vi "Get Vim-formation.vi"(8 "error in (no error)":errorcluster, 9 "ProjectItem Refnum":refnum<vi>, 10 "Path":path, 11 "Map in":map{path, T1}(c390)) -> (0 "error out":errorcluster, 3 "Map out":map{path, T1}(c390))   [LabVIEW 2020, in "vim-liner.lvlib"]
uses:
  vim-liner.lvlib
  vim-formation.ctl
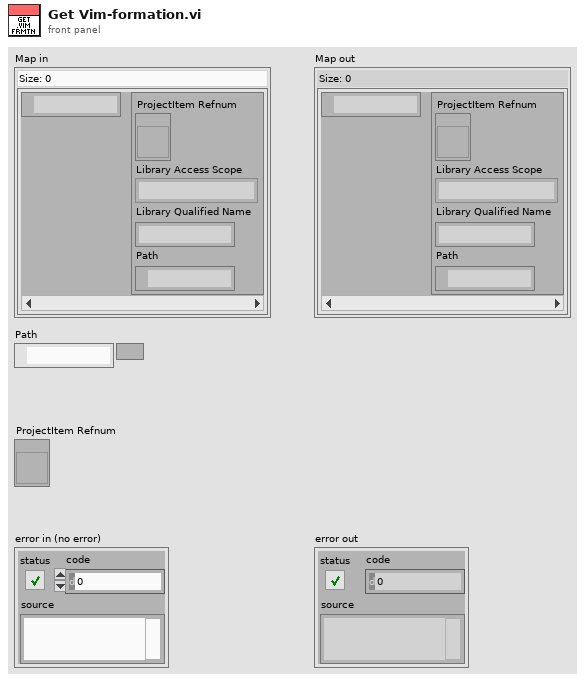
[diagram p1: front panel]
types:
  T1 = typedef "vim-liner.lvlib/vim-formation.ctl" = cluster{"ProjectItem Refnum":refnum<vi>, "Library Access Scope":enum32{"invalid scope", "public", "private", "protected", "community"}, "Library Qualified Name":string, "Path":path}
  T2 = enum32{"invalid scope", "public", "private", "protected", "community"}
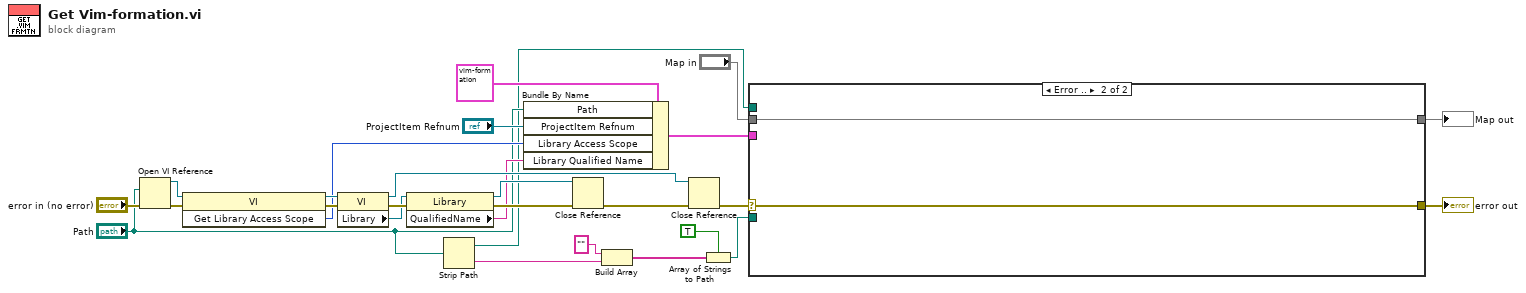
[diagram p0: block diagram]
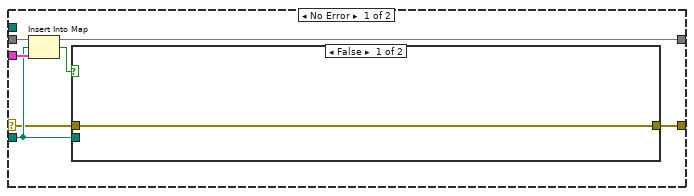
[diagram p2: hidden frame]
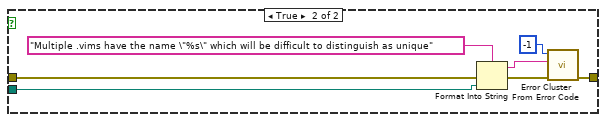
[diagram p3: hidden frame]
diagram:
  n1 = Open VI Reference(vi path="Path", error in (no error)="error in (no error)") -> (vi reference=w18:refnum<vi>, error out=w17:errorcluster)  [unwired: 4 in]
  n2 = invoke class="VI" method="Get Library Access Scope"(reference=w18, error in=w17) -> (reference out=w19:refnum<vi>, error out=w20:errorcluster, "Get Library Access Scope"=w10:T2)  [unwired: 1 in]
  n3 = property class="VI"(reference=w19, error in=w20) -> (reference out=w26:refnum<vi>, error out=w22:errorcluster, "Library"=w21:refnum<vi>)
  n4 = property class="Library"(reference=w21, error in=w22) -> (reference out=w24:refnum<vi>, error out=w23:errorcluster, "QualifiedName"=w9:string)
  n5 = Strip Path(path="Path") -> (stripped path=w7:path, name=w6:string)
  n6 = Bundle By Name(cluster=T1 {"ProjectItem Refnum"=refnum, "Library Access Scope"=enum."invalid scope", "Library Qualified Name"="", "Path"=path ""} (".vim"), "Path"="Path", "ProjectItem Refnum"="ProjectItem Refnum", "Library Access Scope"=w10, "Library Qualified Name"=w9) -> (w13:T1)
  n7 = Close Reference(reference=w24, error in (no error)=w23) -> (error out=w25:errorcluster)
  n8 = Build Array("" ("element"), w6) -> (w5:string[])
  n9 = Close Reference(reference=w26, error in (no error)=w25) -> (error out=w14:errorcluster)
  n10 = Array of Strings to Path(0:w5, 1:TRUE ("relative")) -> (2:w2:path)
  n11 = case shown="Error .." w14 {
    selector: w14 -> [w29 w43]
    tunnel: w13 -> [w34 _]
    tunnel: w7 -> [_ _]
    tunnel: "Map in" -> [w33 w44]
    tunnel: [w32 w44] -> w11
    tunnel: w2 -> [w30 _]
    tunnel: [w28 w43] -> w1
    frame No Error {
      n12 = Insert Into Map(map in=w33, key=w30, value=w34) -> (map out=w32:map{path, T1}, key already included?=w31:bool)  [unwired: 1 out]
      n13 = case shown="False" w31 {
        tunnel: w30 -> [_ w42]
        tunnel: w29 -> [w35 w37]
        tunnel: [w35 w36] -> w28
        frame False {
        }
        frame True {
          n14 = Format Into String(format string="Multiple .vims have the name \"%s\" which will be difficult to distinguish as unique", error in=w37, w42) -> (resulting string=w39:string, error out=w40:errorcluster)  [unwired: 1 in]
          n15 = call <vilib>:"Error Cluster From Error Code.vi"("error in (no error)"=w40, "error message (\"\")"=w39, "error code (0)"=-1) -> ("error out"=w36:errorcluster)  [unwired: 6 in]
        }
      }
    }
    frame Error {
    }
  }
  "Map out" <- w11
  "error out" <- w1
